vi "Open_Close_Front_Panel.ph.vi"(2 "Front Panel Window:Open":bool=TRUE, 3 "VI path":path) -> (0 "error out":errorcluster)   [LabVIEW 2017]
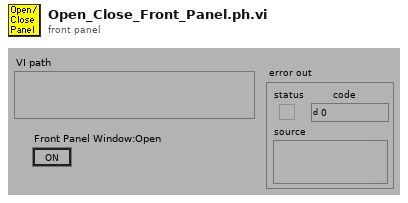
[diagram p1: front panel]
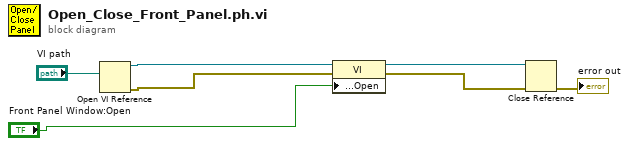
[diagram p0: block diagram]
diagram:
  n1 = Open VI Reference(vi path="VI path") -> (vi reference=w4:refnum<vi>, error out=w3:errorcluster)  [unwired: 1 in, 4 out]
  n2 = property class="VI"(reference=w4, error in=w3, "Front Panel Window:Open"="Front Panel Window:Open") -> (reference out=w2:refnum<vi>, error out=w1:errorcluster)
  n3 = Close Reference(reference=w2, error in (no error)=w1) -> (error out=→"error out":errorcluster)
